vi "油压显示.vi"(0 "WaveformGraph输入":refnum<vi>, 4 "F":dbl, 5 "F1":dbl, 8 "x+y":dbl, 9 "F2":dbl, 13 "V2":dbl, 15 "V1":dbl) -> ()   [LabVIEW 2011]
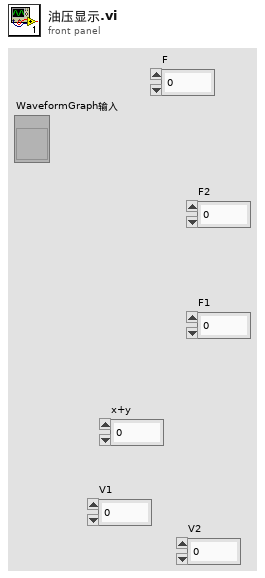
[diagram p1: front panel]
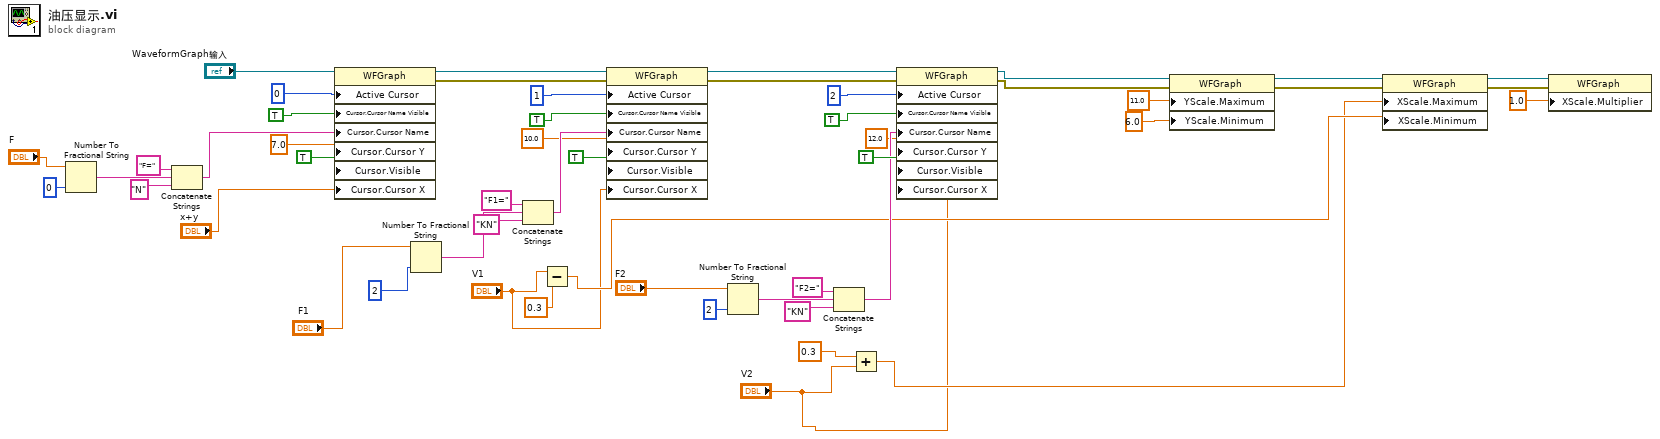
[diagram p0: block diagram]
diagram:
  n1 = Number To Fractional String(number="F", precision (6)=i16 0 ("精度(6)")) -> (F-format string=w16:string)  [unwired: 2 in]
  n2 = Concatenate Strings("F=" ("字符串"), w16, "N" ("字符串")) -> (w13:string)
  n3 = property on="属性节点" class="WFGraph"(reference="WaveformGraph输入", "Active Cursor"=u32 0 ("活动游标"), "Cursor.Cursor Name Visible"=TRUE ("光标.游标名可见"), "Cursor.Cursor Name"=w13, "Cursor.Cursor Y"=7.0 ("光标.游标位置:游标Y坐标"), "Cursor.Visible"=TRUE ("光标.可见"), "Cursor.Cursor X"="x+y") -> (reference out=w41:refnum<vi>, error out=w31:errorcluster)  [unwired: 1 in]
  n4 = Number To Fractional String(number="F1", precision (6)=i16 2 ("宽度(-)")) -> (F-format string=w29:string)  [unwired: 2 in]
  n5 = Concatenate Strings("F1=" ("字符串"), w29, "KN" ("字符串")) -> (w25:string)
  n6 = Subtract(x="V1", y=0.3 ("x")) -> (x-y=w6:dbl)
  n7 = property on="属性节点" class="WFGraph"(reference=w41, error in=w31, "Active Cursor"=u32 1 ("活动游标"), "Cursor.Cursor Name Visible"=TRUE ("光标.游标名可见"), "Cursor.Cursor Name"=w25, "Cursor.Cursor Y"=10.0 ("光标.游标位置:游标Y坐标"), "Cursor.Visible"=TRUE ("光标.可见"), "Cursor.Cursor X"="V1") -> (reference out=w42:refnum<vi>, error out=w43:errorcluster)
  n8 = Number To Fractional String(number="F2", precision (6)=i16 2 ("宽度(-)")) -> (F-format string=w21:string)  [unwired: 2 in]
  n9 = Concatenate Strings("F2=" ("字符串"), w21, "KN" ("字符串")) -> (w19:string)
  n10 = Add(x=0.3, y="V2") -> (x+y=w4:dbl)
  n11 = property on="属性节点" class="WFGraph"(reference=w42, error in=w43, "Active Cursor"=u32 2 ("活动游标"), "Cursor.Cursor Name Visible"=TRUE ("光标.游标名可见"), "Cursor.Cursor Name"=w19, "Cursor.Cursor Y"=12.0 ("光标.游标位置:游标Y坐标"), "Cursor.Visible"=TRUE ("光标.可见"), "Cursor.Cursor X"="V2") -> (reference out=w12:refnum<vi>, error out=w11:errorcluster)
  n12 = property on="属性节点" class="WFGraph"(reference=w12, error in=w11, "YScale.Maximum"=11.0 ("Y标尺.范围:最大值"), "YScale.Minimum"=6.0 ("Y标尺.范围:最小值")) -> (reference out=w48:refnum<vi>, error out=w45:errorcluster)
  n13 = property on="属性节点" class="WFGraph"(reference=w48, error in=w45, "XScale.Maximum"=w4, "XScale.Minimum"=w6) -> (reference out=w49:refnum<vi>, error out=w50:errorcluster)
  n14 = property on="属性节点" class="WFGraph"(reference=w49, error in=w50, "XScale.Multiplier"=1.0 ("X标尺.偏移量与缩放系数:缩放系数")) -> ()  [unwired: 2 out]
